vi "Describe Variant.vi"(11 "Variant":variant) -> (1 "Type Description":string, 2 "Description":string, 3 "Variant Description":string)   [LabVIEW 2020, in "Utilities.lvlib"]
uses:
  Utilities.lvlib
  <vilib>/Utility/Data Type/NI_Data Type.lvlib
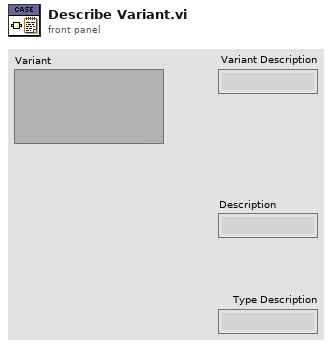
[diagram p1: front panel]
types:
  T1 = typedef "NI_Data Type.lvlib/Data Type.ctl" = enum8{"Invalid Type", "Void", "I8", "I16", "I32", "I64", "U8", "U16", "U32", "U64", "Single Float", "Double Float", "Extended Float", "Single Complex", "Double Complex", "Extended Complex", "Enum U8", "Enum U16", "Enum U32", "Enum U64", "Single Float With Unit", "Double Float With Unit", "Extended Float With Unit", "Single Complex with Unit", "Double Complex with Unit", "Extended Complex with Unit", "Boolean", "String", "Path", "Picture", "Tag", "Array", "Cluster", "Variant", "LV Variant", "Waveform", "Timestamp", "Digital Waveform", "Digital Data", "ExpressData", "Refnum", "External Data", "VI", "Poly VI", "LabVIEW Class Instance", "Fixed Point", "Set Collection", "Map Collection"}
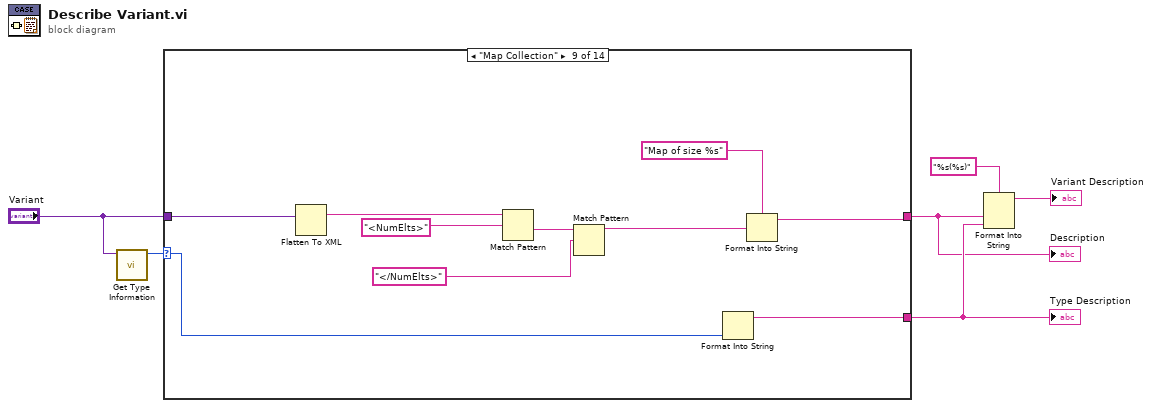
[diagram p0: block diagram]
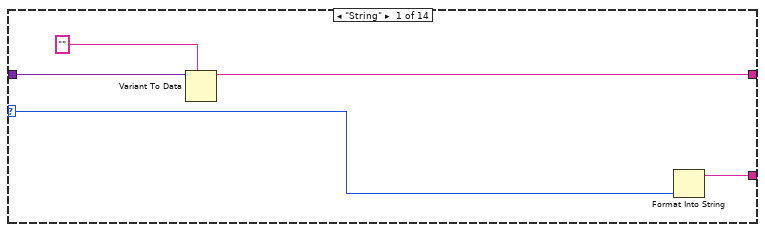
[diagram p2: hidden frame]
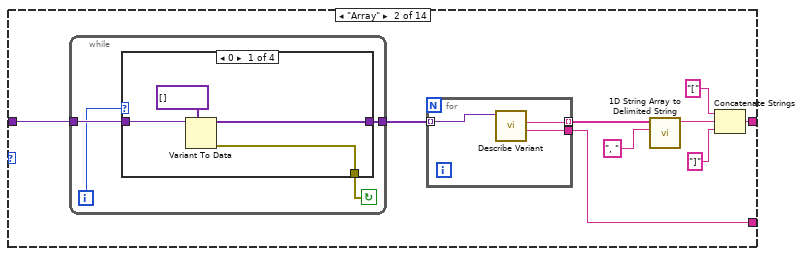
[diagram p3: hidden frame]
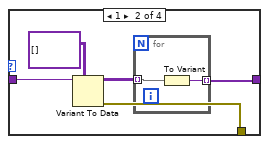
[diagram p4: hidden frame]
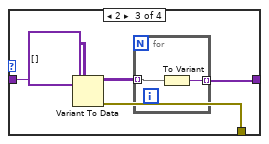
[diagram p5: hidden frame]
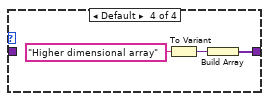
[diagram p6: hidden frame]
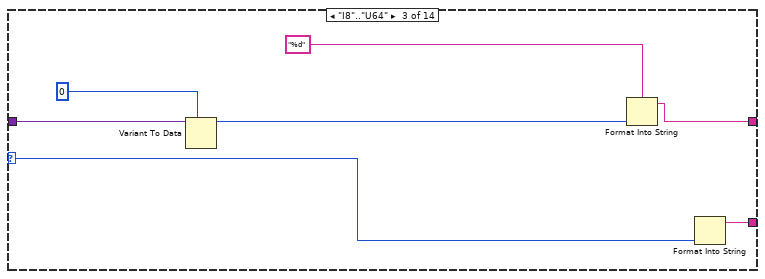
[diagram p7: hidden frame]
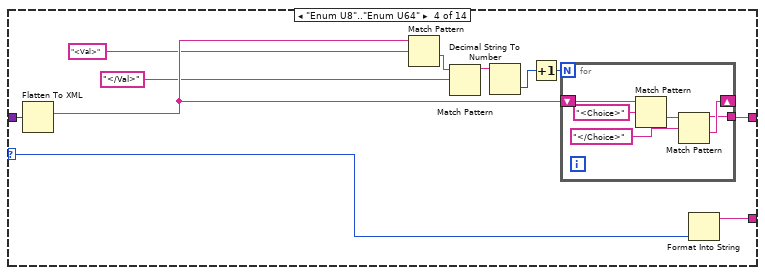
[diagram p8: hidden frame]
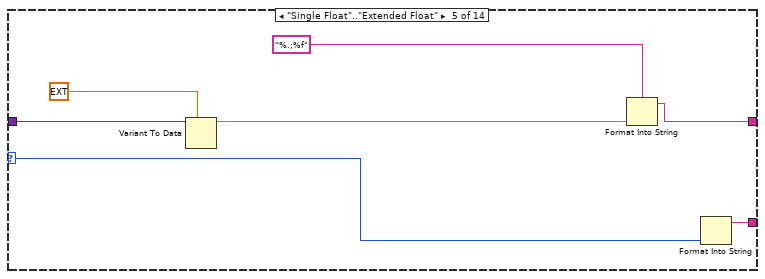
[diagram p9: hidden frame]
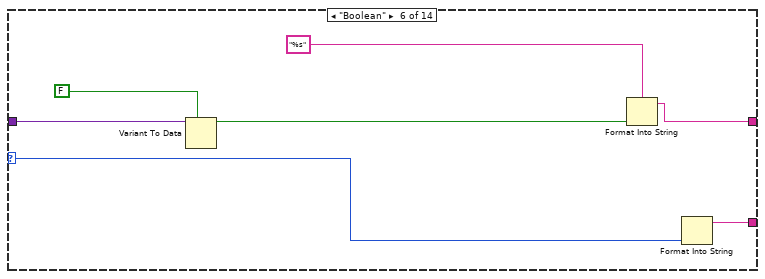
[diagram p10: hidden frame]
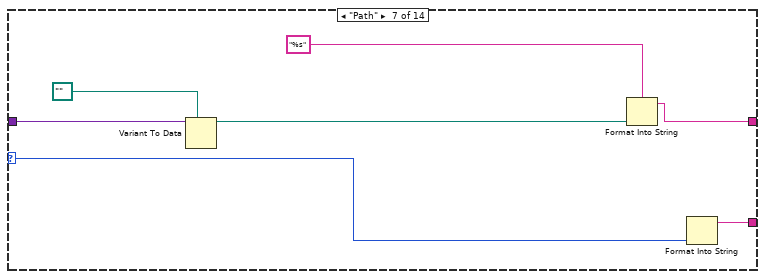
[diagram p11: hidden frame]
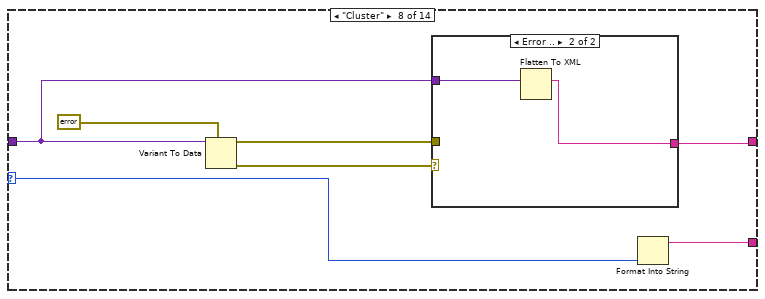
[diagram p12: hidden frame]
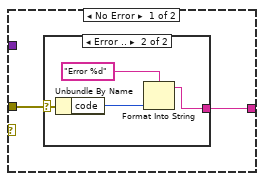
[diagram p13: hidden frame]
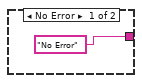
[diagram p14: hidden frame]
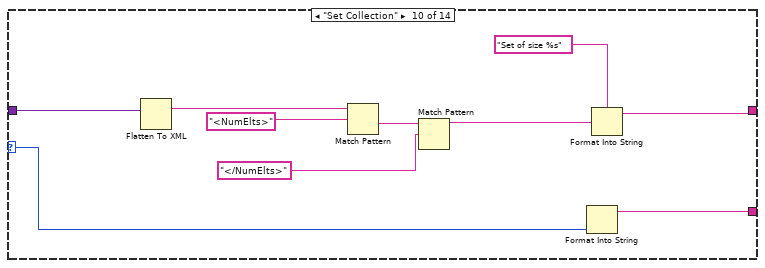
[diagram p15: hidden frame]
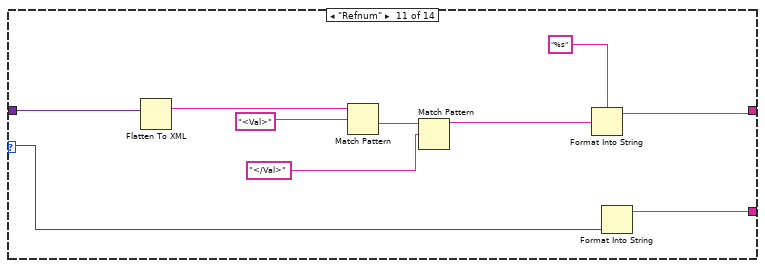
[diagram p16: hidden frame]
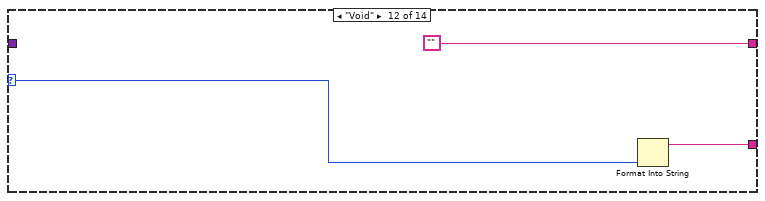
[diagram p17: hidden frame]
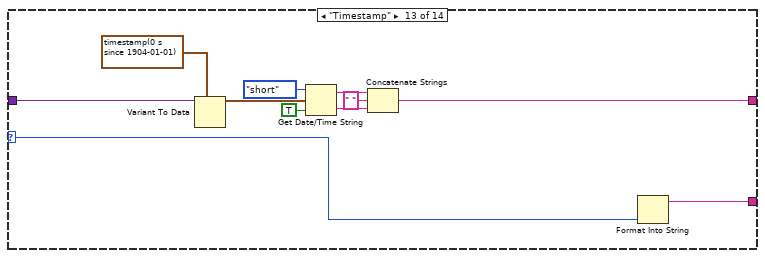
[diagram p18: hidden frame]
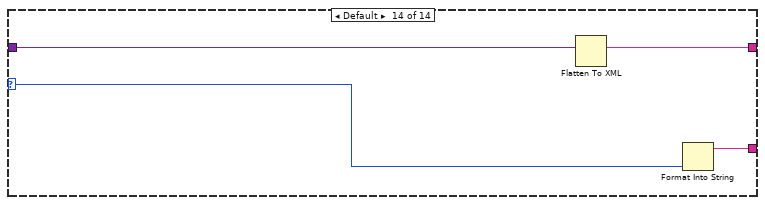
[diagram p19: hidden frame]
diagram:
  n1 = call <vilib>:"Get Type Information.vi"("variant"="Variant") -> ("type"=w5:T1)  [unwired: 6 in, 4 out]
  n2 = case shown="\"Map Collection\"" w5 {
    selector: w5 -> [w7 _ w49 w65 w73 w80 w87 w98 w110 w120 w130 w142 w153 w154]
    tunnel: "Variant" -> [w11 w20 w55 w57 w79 w86 w93 w94 w119 w129 w139 _ w151 w157]
    tunnel: [w10 w15 w51 w56 w75 w82 w89 w96 w112 w122 w132 "" w143 w156] -> w2
    tunnel: [w8 w12 w50 w66 w74 w81 w88 w97 w111 w121 w131 w141 w152 w155] -> w4
    frame "String" {
      n3 = Variant To Data(type="", Variant=w11) -> (data=w10:string)  [unwired: 1 in, 1 out]
      n4 = Format Into String(w7) -> (resulting string=w8:string)  [unwired: 3 in, 1 out]
    }
    frame "Array" {
      n5 = while {
        tunnel: w20 -> [w24]
        tunnel: [w23] -> w19
        i -> [w22]
        stop <- w21 continue-if-true
        n6 = case shown="0" w22 {
          tunnel: w24 -> [w28 w33 w40 _]
          tunnel: [w26 w30 w37 w43] -> w23
          tunnel: [w25 w29 w36 _] -> w21
          frame 0 {
            n7 = Variant To Data(type=variant[] [], Variant=w28) -> (data=w26:variant[], error out=w25:errorcluster)  [unwired: 1 in]
          }
          frame 1 {
            n8 = Variant To Data(type=variant[][] [], Variant=w33) -> (data=w31:variant[][], error out=w29:errorcluster)  [unwired: 1 in]
            n9 = for {
              tunnel: w31 -> [w35] mode=indexing
              tunnel: [w34] -> w30 mode=indexing
              n10 = To Variant(anything=w35) -> (Variant=w34:variant)
            }
          }
          frame 2 {
            n11 = Variant To Data(type=variant[][][] [], Variant=w40) -> (data=w38:variant[][][], error out=w36:errorcluster)  [unwired: 1 in]
            n12 = for {
              tunnel: w38 -> [w42] mode=indexing
              tunnel: [w41] -> w37 mode=indexing
              n13 = To Variant(anything=w42) -> (Variant=w41:variant)
            }
          }
          frame Default {
            n14 = To Variant(anything="Higher dimensional array") -> (Variant=w44:variant)
            n15 = Build Array(w44) -> (w43:variant[])
          }
        }
      }
      n16 = for {
        tunnel: w19 -> [w48] mode=indexing
        tunnel: [w46] -> w17 mode=indexing
        tunnel: [w47] -> w12
        n17 = call "Describe Variant.vi"("Variant"=w48) -> ("Type Description"=w47:string, "Description"=w46:string)  [unwired: 8 in, 1 out]
      }
      n18 = call <vilib>:"1D String Array to Delimited String.vi"("delimiter"=", ", "string array"=w17) -> ("delimited string"=w16:string)  [unwired: 9 in]
      n19 = Concatenate Strings("[", w16, "]") -> (w15:string)
    }
    frame "I8".."U64" {
      n20 = Variant To Data(type=i64 0, Variant=w55) -> (data=w53:i64)  [unwired: 1 in, 1 out]
      n21 = Format Into String(format string="%d", w53) -> (resulting string=w51:string)  [unwired: 2 in, 1 out]
      n22 = Format Into String(w49) -> (resulting string=w50:string)  [unwired: 3 in, 1 out]
    }
    frame "Enum U8".."Enum U64" {
      n23 = Flatten To XML(6:w57) -> (2:w60:string)
      n24 = Match Pattern(string=w60, regular expression="<Val>" ("string")) -> (after substring=w61:string)  [unwired: 1 in, 3 out]
      n25 = Match Pattern(string=w61, regular expression="</Val>") -> (before substring=w62:string)  [unwired: 1 in, 3 out]
      n26 = Decimal String To Number(string=w62) -> (number=w63:i32)  [unwired: 2 in, 1 out]
      n27 = Increment(x=w63) -> (x+1=w64:i32)
      n28 = for {
        N: w64 -> [_]
        shift-right: [w68] -> _
        shift-left: w60 -> [w70]
        tunnel: [w67] -> w56
        n29 = Match Pattern(string=w70, regular expression="<Choice>" ("string")) -> (after substring=w72:string)  [unwired: 1 in, 3 out]
        n30 = Match Pattern(string=w72, regular expression="</Choice>") -> (before substring=w67:string, after substring=w68:string)  [unwired: 1 in, 2 out]
      }
      n31 = Format Into String(w65) -> (resulting string=w66:string)  [unwired: 3 in, 1 out]
    }
    frame "Single Float".."Extended Float" {
      n32 = Variant To Data(type=ext 0.0, Variant=w79) -> (data=w77:ext)  [unwired: 1 in, 1 out]
      n33 = Format Into String(format string="%.;%f", w77) -> (resulting string=w75:string)  [unwired: 2 in, 1 out]
      n34 = Format Into String(w73) -> (resulting string=w74:string)  [unwired: 3 in, 1 out]
    }
    frame "Boolean" {
      n35 = Variant To Data(type=FALSE, Variant=w86) -> (data=w84:bool)  [unwired: 1 in, 1 out]
      n36 = Format Into String(format string="%s", w84) -> (resulting string=w82:string)  [unwired: 2 in, 1 out]
      n37 = Format Into String(w80) -> (resulting string=w81:string)  [unwired: 3 in, 1 out]
    }
    frame "Path" {
      n38 = Variant To Data(type=path "", Variant=w93) -> (data=w91:path)  [unwired: 1 in, 1 out]
      n39 = Format Into String(format string="%s", w91) -> (resulting string=w89:string)  [unwired: 2 in, 1 out]
      n40 = Format Into String(w87) -> (resulting string=w88:string)  [unwired: 3 in, 1 out]
    }
    frame "Cluster" {
      n41 = Variant To Data(type=errorcluster {"status"=FALSE, "code"=0, "source"=""} ("error in"), Variant=w94) -> (data=w99:errorcluster, error out=w95:errorcluster)  [unwired: 1 in]
      n42 = case shown="Error .." w95 {
        tunnel: w99 -> [w102 _]
        tunnel: [w101 w108] -> w96
        tunnel: w94 -> [_ w109]
        frame No Error {
          n43 = case shown="Error .." w102 {
            selector: w102 -> [_ w107]
            tunnel: ["No Error" w105] -> w101
            frame No Error {
            }
            frame Error {
              n44 = Unbundle By Name(w107) -> ("code"=w106:i32)
              n45 = Format Into String(format string="Error %d", w106) -> (resulting string=w105:string)  [unwired: 2 in, 1 out]
            }
          }
        }
        frame Error {
          n46 = Flatten To XML(6:w109) -> (2:w108:string)
        }
      }
      n47 = Format Into String(w98) -> (resulting string=w97:string)  [unwired: 3 in, 1 out]
    }
    frame "Map Collection" {
      n48 = Flatten To XML(6:w119) -> (2:w114:string)
      n49 = Match Pattern(string=w114, regular expression="<NumElts>" ("string")) -> (after substring=w117:string)  [unwired: 1 in, 3 out]
      n50 = Match Pattern(string=w117, regular expression="</NumElts>" ("string")) -> (before substring=w115:string)  [unwired: 1 in, 3 out]
      n51 = Format Into String(w110) -> (resulting string=w111:string)  [unwired: 3 in, 1 out]
      n52 = Format Into String(format string="Map of size %s", w115) -> (resulting string=w112:string)  [unwired: 2 in, 1 out]
    }
    frame "Set Collection" {
      n53 = Flatten To XML(6:w129) -> (2:w124:string)
      n54 = Match Pattern(string=w124, regular expression="<NumElts>" ("string")) -> (after substring=w127:string)  [unwired: 1 in, 3 out]
      n55 = Match Pattern(string=w127, regular expression="</NumElts>" ("string")) -> (before substring=w125:string)  [unwired: 1 in, 3 out]
      n56 = Format Into String(w120) -> (resulting string=w121:string)  [unwired: 3 in, 1 out]
      n57 = Format Into String(format string="Set of size %s", w125) -> (resulting string=w122:string)  [unwired: 2 in, 1 out]
    }
    frame "Refnum" {
      n58 = Flatten To XML(6:w139) -> (2:w134:string)
      n59 = Match Pattern(string=w134, regular expression="<Val>" ("string")) -> (after substring=w137:string)  [unwired: 1 in, 3 out]
      n60 = Match Pattern(string=w137, regular expression="</Val>" ("string")) -> (before substring=w135:string)  [unwired: 1 in, 3 out]
      n61 = Format Into String(format string="%s", w135) -> (resulting string=w132:string)  [unwired: 2 in, 1 out]
      n62 = Format Into String(w130) -> (resulting string=w131:string)  [unwired: 3 in, 1 out]
    }
    frame "Void" {
      n63 = Format Into String(w142) -> (resulting string=w141:string)  [unwired: 3 in, 1 out]
    }
    frame "Timestamp" {
      n64 = Variant To Data(type=timestamp(0 s since 1904-01-01) ("current time"), Variant=w151) -> (data=w149:timestamp)  [unwired: 1 in, 1 out]
      n65 = Get Date/Time String(date format (0)=enum16{"short", "long", "abbreviated"}."short", seconds (now)=w149, want seconds? (F)=TRUE) -> (date string=w146:string, time string=w145:string)
      n66 = Concatenate Strings(w146, " " ("string"), w145) -> (w143:string)
      n67 = Format Into String(w153) -> (resulting string=w152:string)  [unwired: 3 in, 1 out]
    }
    frame Default {
      n68 = Flatten To XML(6:w157) -> (2:w156:string)
      n69 = Format Into String(w154) -> (resulting string=w155:string)  [unwired: 3 in, 1 out]
    }
  }
  "Type Description" <- w4
  "Description" <- w2
  n70 = Format Into String(format string="%s(%s)", w2, w4) -> (resulting string=→"Variant Description":string)  [unwired: 2 in, 1 out]
